vi "Zero Crossing.vi"(0 "waveforms in":waveform(dbl)[](array[waveform]), 1 "reset? (F)":bool, 7 "nominal sampling rate":dbl, 11 "error in":errorcluster) -> (4 "waveforms out":waveform(dbl)[](array[waveform]), 6 "zero crossings":cluster{"zero crossing":dbl[]}[](array[cluster]), 8 "samples since the last cross":cluster{"samples since the last cross":dbl[]}[](array[cluster]), 15 "error out":errorcluster)   [LabVIEW 2016]
doc: "Calculates the zero crossing indexes for voltage waveforms, current waveforms, or waveforms that contain both voltage and current. Zero crossing is the instantaneous point at which the voltage or current turns from positive to negative or from negative to positive.\n\nThis VI supports measuring single-line and multiple-line systems."
uses:
  <vilib>/addons/Electrical Power/PQ/NI_EP_Power Quality.lvlib
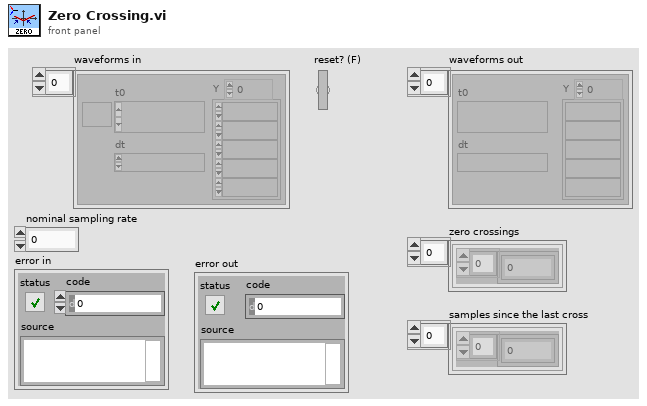
[diagram p1: front panel]
types:
  T1 = cluster{"filter structure":enum32{"IIR 2nd Order", "IIR 4th Order"}, "Reverse Coefficients":dbl[], "Forward Coefficients":dbl[]}
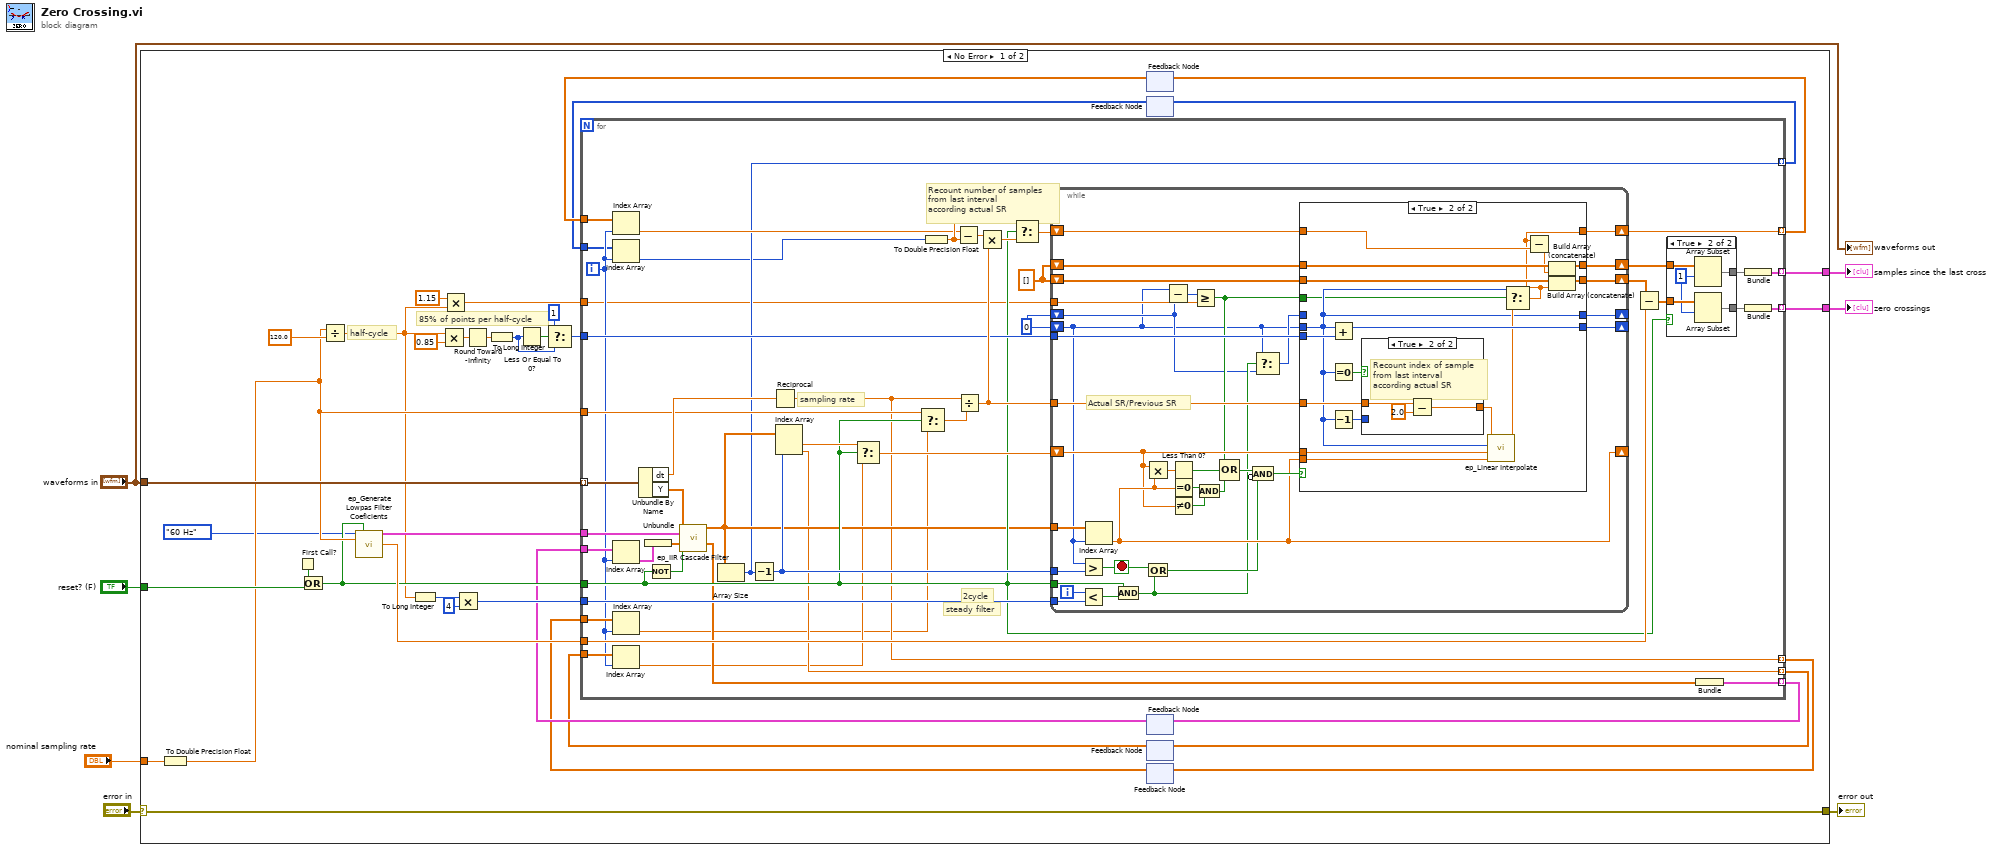
[diagram p0: block diagram]
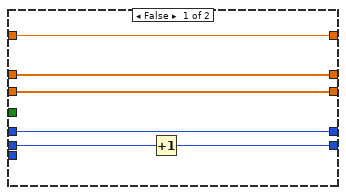
[diagram p3: hidden frame]
diagram:
  n1 = case shown="No Error" "error in" {
    selector: "error in" -> [w8 w161]
    tunnel: "waveforms in" -> [w43 _]
    tunnel: [w38 _] -> w7
    tunnel: [w37 _] -> w6
    tunnel: [w8 w161] -> w1
    tunnel: "reset? (F)" -> [w30 _]
    tunnel: "nominal sampling rate" -> [w9 _]
    frame No Error {
      # "85% of points per half-cycle"
      # "half-cycle"
      n2 = To Double Precision Float(number=w9) -> (double precision float=w25:dbl)
      n3 = First Call?() -> (First Call?: T/F=w29:bool)
      n4 = Or(x=w29, y=w30) -> (x .or. y?=w24:bool)
      n5 = Divide(x=w25, y=120.0) -> (x/y=w12:dbl)
      n6 = call <vilib>:"ep_Generate Lowpas Filter Coeficients.vi"("nominal frequency"=enum16{"50 Hz", "60 Hz"}."60 Hz", "restart (F)"=w24, "nominal sampling rate (Hz)"=w25) -> ("IIR filter cluster"=w36:T1, "filter delay (samples)"=w35:dbl)  [unwired: 11 in]
      n7 = To Long Integer(number=w12) -> (32bit integer=w39:i32)
      n8 = Multiply(x=w12, y=0.85) -> (x*y=w28:dbl)
      n9 = Multiply(x=1.15 ("y"), y=w12) -> (x*y=w11:dbl)
      n10 = Multiply(x=w39, y=4) -> (x*y=w41:i32)
      n11 = Round Toward -Infinity(1:w28) -> (0:w26:dbl)
      n12 = To Long Integer(number=w26) -> (32bit integer=w31:i32)
      n13 = Less Or Equal To 0?(x=w31) -> (x <= 0?=w34:bool)
      n14 = Select(t=1, s=w34, f=w31) -> (s? t:f=w32:i32)
      n15 = feedback #1() -> (w22:dbl[])  [unwired: 1 in]
      n16 = feedback #2() -> (w14:i32[])  [unwired: 1 in]
      n17 = feedback #3() -> (w20:cluster{"shift register out":dbl[]}[])  [unwired: 1 in]
      n18 = feedback #4() -> (w18:dbl[])  [unwired: 1 in]
      n19 = feedback #5() -> (w16:dbl[])  [unwired: 1 in]
      n20 = for {
        tunnel: w43 -> [w90] mode=indexing
        tunnel: w41 -> [w87]
        tunnel: [w69] -> w38 mode=indexing
        tunnel: [w68] -> w37 mode=indexing
        tunnel: w36 -> [w65]
        tunnel: w35 -> [w84]
        tunnel: w32 -> [w83]
        tunnel: w25 -> [w71]
        tunnel: w24 -> [w70]
        tunnel: [w67] -> w23 mode=indexing
        tunnel: w22 -> [w62]
        tunnel: w20 -> [w58]
        tunnel: [w59] -> w21 mode=indexing
        tunnel: [w55] -> w19 mode=indexing
        tunnel: w18 -> [w54]
        tunnel: [w52] -> w17 mode=indexing
        tunnel: w16 -> [w51]
        tunnel: [w49] -> w15 mode=indexing
        tunnel: w14 -> [w47]
        tunnel: w11 -> [w44]
        i -> [w48]
        w79 = dbl[] []
        w45 = 0
        # "Recount number of samples\nfrom last interval\naccording actual SR"
        # "steady filter"
        # "2cycle"
        # "sampling rate"
        n21 = Index Array(array=w62, index=w48) -> (element=w61:dbl)
        n22 = Index Array(array=w47, index=w48) -> (element=w46:i32)
        n23 = Index Array(array=w58, index=w48) -> (element=w57:cluster{"shift register out":dbl[]})
        n24 = Index Array(array=w51, index=w48) -> (element=w50:dbl)
        n25 = Index Array(array=w54, index=w48) -> (element=w53:dbl)
        n26 = Unbundle By Name(w90) -> ("dt"=w89:dbl, "Y"=w63:dbl[])
        n27 = Unbundle(w57) -> ("shift register out"=w56:dbl[])
        n28 = Not(x=w70) -> (.not. x?=w64:bool)
        n29 = call <vilib>:"ep_IIR Cascade Filter.vi"("X"=w63, "IIR Filter Cluster"=w65, "shift register in"=w56, "init/cont (init:F)"=w64) -> ("Filtered X"=w66:dbl[], "shift register out"=w60:dbl[])  [unwired: 9 in, 1 out]
        n30 = Array Size(array=w66) -> (size(s)=w49:i32)
        n31 = Decrement(x=w49) -> (x-1=w91:i32)
        n32 = Reciprocal(x=w89) -> (1/x=w52:dbl)
        n33 = Index Array(array=w66, index #2=w91) -> (element #1=w81:dbl, element #2=w55:dbl)  [unwired: 1 in]
        n34 = Select(t=w81, s=w70, f=w53) -> (s? t:f=w82:dbl)
        n35 = Select(t=w71, s=w70, f=w50) -> (s? t:f=w80:dbl)
        n36 = To Double Precision Float(number=w46) -> (double precision float=w72:dbl)
        n37 = Subtract(x=w61, y=w72) -> (x-y=w78:dbl)
        n38 = Divide(x=w52, y=w80) -> (x/y=w88:dbl)
        n39 = Multiply(x=w78, y=w88) -> (x*y=w74:dbl)
        n40 = Select(t=w72, s=w70, f=w74) -> (s? t:f=w73:dbl)
        n41 = while {
          shift-right: [w131] -> w75
          shift-left: w79 -> [w129]
          shift-right: [w125] -> _
          shift-left: w82 -> [w107]
          tunnel: w66 -> [w132]
          tunnel: w91 -> [w127]
          shift-right: [w130] -> _
          shift-left: w45 -> [w99]
          tunnel: w83 -> [w128]
          tunnel: w88 -> [w124]
          shift-right: [w123] -> w67
          shift-left: w73 -> [w122]
          shift-right: [w120] -> w77
          shift-left: w79 -> [w121]
          tunnel: w70 -> [w117]
          tunnel: w87 -> [w115]
          shift-right: [w104] -> _
          shift-left: w45 -> [w100]
          tunnel: w44 -> [w105]
          i -> [w116]
          stop <- w119 stop-if-true
          # "Actual SR/Previous SR"
          n42 = Greater?(x=w99, y=w127) -> (0:w119:bool)
          n43 = Less?(x=w116, y=w115) -> (x < y?=w118:bool)
          n44 = Index Array(array=w132, index=w99) -> (element=w125:dbl)
          n45 = And(x=w117, y=w118) -> (x .and. y?=w102:bool)
          n46 = Multiply(x=w107, y=w125) -> (x*y=w114:dbl)
          n47 = Or(x=w119, y=w102) -> (x .or. y?=w108:bool)
          n48 = Subtract(x=w99, y=w100) -> (x-y=w106:i32)
          n49 = Less Than 0?(x=w114) -> (x < 0?=w111:bool)
          n50 = Equal To 0?(x=w125) -> (x = 0?=w113:bool)
          n51 = Not Equal To 0?(x=w107) -> (x != 0?=w112:bool)
          n52 = Greater Or Equal?(x=w106, y=w105) -> (x >= y?=w103:bool)
          n53 = And(x=w113, y=w112) -> (x .and. y?=w110:bool)
          n54 = Compound Arithmetic op=OR(w103, w111, w110) -> (w109:bool)
          n55 = Compound Arithmetic op=AND(w109, invert w108) -> (w126:bool)
          n56 = Select(t=w99, s=w102, f=w100) -> (s? t:f=w101:i32)
          n57 = case shown="True" w126 {
            tunnel: w129 -> [w138 w156]
            tunnel: [w138 w155] -> w131
            tunnel: w99 -> [w137 w140]
            tunnel: [w136 w149] -> w130
            tunnel: w128 -> [_ w154]
            tunnel: w107 -> [_ w153]
            tunnel: w125 -> [_ w152]
            tunnel: w124 -> [_ w148]
            tunnel: [w135 w141] -> w123
            tunnel: w122 -> [w135 w147]
            tunnel: w121 -> [w134 w146]
            tunnel: [w134 w144] -> w120
            tunnel: w103 -> [_ w139]
            tunnel: w101 -> [w133 _]
            tunnel: [w133 w140] -> w104
            frame False {
              n58 = Increment(x=w137) -> (x+1=w136:i32)
            }
            frame True {
              n59 = Add(x=w140, y=w154) -> (x+y=w149:i32)
              n60 = Equal To 0?(x=w140) -> (x = 0?=w151:bool)
              n61 = Decrement(x=w140) -> (x-1=w150:i32)
              n62 = case shown="True" w151 {
                tunnel: w150 -> [w157 _]
                tunnel: [w157 w158] -> w143
                tunnel: w148 -> [_ w160]
                frame False {
                }
                frame True {
                  # "Recount index of sample\nfrom last interval\naccording actual SR"
                  n63 = Subtract(x=w160, y=2.0) -> (x-y=w158:dbl)
                }
              }
              n64 = call <vilib>:"ep_Linear Interpolate.vi"("y2"=w152, "y1"=w153, "x2"=w140, "x1"=w143) -> ("y"=w142:dbl)  [unwired: 7 in]
              n65 = Select(t=w140, s=w139, f=w142) -> (s? t:f=w141:dbl)
              n66 = Subtract(x=w141, y=w147) -> (x-y=w145:dbl)
              n67 = Build Array (concatenate)(w146, w145) -> (w144:dbl[])
              n68 = Build Array (concatenate)(w156, w141) -> (w155:dbl[])
            }
          }
        }
        n69 = Subtract(x=w75, y=w84) -> (x-y=w76:dbl[])
        n70 = case shown="True" w70 {
          tunnel: w77 -> [w92 w98]
          tunnel: [w92 w97] -> w86
          tunnel: w76 -> [w93 w96]
          tunnel: [w93 w95] -> w85
          frame False {
          }
          frame True {
            w94 = 1 ("index")
            n71 = Array Subset(array=w98, index=w94) -> (w97:dbl[])  [unwired: 1 in]
            n72 = Array Subset(array=w96, index=w94) -> (w95:dbl[])  [unwired: 1 in]
          }
        }
        n73 = Bundle("shift register out"=w60) -> (w59:cluster{"shift register out":dbl[]})  [unwired: 1 in]
        n74 = Bundle(w86) -> (w69:cluster{dbl[]})  [unwired: 1 in]
        n75 = Bundle(w85) -> (w68:cluster{dbl[]})  [unwired: 1 in]
      }
      n76 = feedback-in #1(w23) -> ()
      n77 = feedback-in #2(w15) -> ()
      n78 = feedback-in #3(w21) -> ()
      n79 = feedback-in #4(w19) -> ()
      n80 = feedback-in #5(w17) -> ()
    }
    frame Error {
    }
  }
  "zero crossings" <- w6
  "samples since the last cross" <- w7
  "error out" <- w1
  "waveforms out" <- "waveforms in"
